vi "RUSHShoot.vi"(1 "In Cluster":T2) -> (0 "Out Cluster":T1)   [LabVIEW 2012]
panel:
  in  "Speed Multiplier":dbl=0.75
  in  "LinReg Adder":dbl=-0.5
  in  "LinReg Multiplier":dbl=0.01
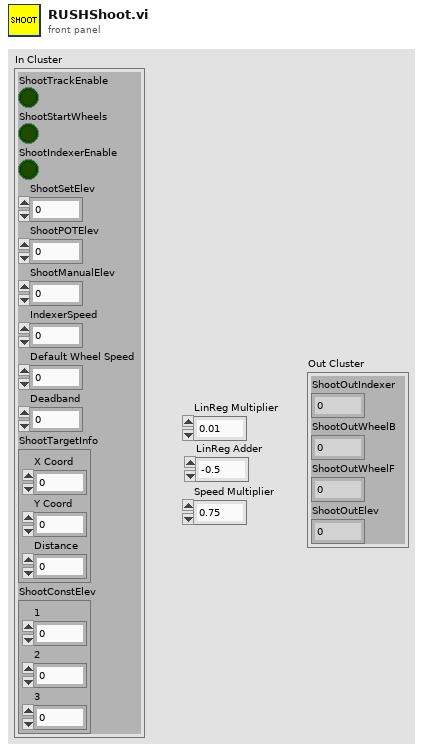
[diagram p1: front panel]
types:
  T1 = cluster{"ShootOutIndexer":dbl, "ShootOutWheelB":dbl, "ShootOutWheelF":dbl, "ShootOutElev":dbl}
  T2 = cluster{"ShootTrackEnable":bool, "ShootStartWheels":bool, "ShootIndexerEnable":bool, "ShootSetElev":dbl, "ShootPOTElev":dbl, "ShootManualElev":dbl, "IndexerSpeed":dbl, "Default Wheel Speed":dbl, "Deadband":dbl, "ShootTargetInfo":cluster{"X Coord":dbl, "Y Coord":dbl, "Distance":dbl}, "ShootConstElev":cluster{"1":dbl, "2":dbl, "3":dbl}}
  T3 = cluster{"X Coord":dbl, "Y Coord":dbl, "Distance":dbl}
  T4 = cluster{"ShootOutIndexer":dbl, "ShootOutWheelB":dbl, "ShootOutWheelF":dbl, "upper limit":dbl}
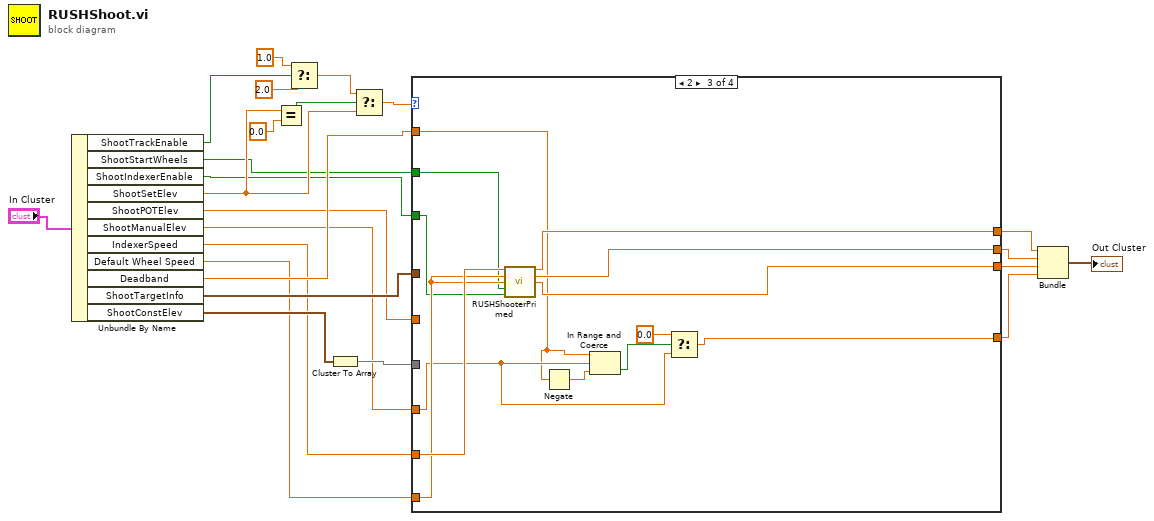
[diagram p0: block diagram]
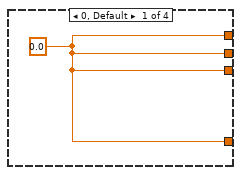
[diagram p2: hidden frame]
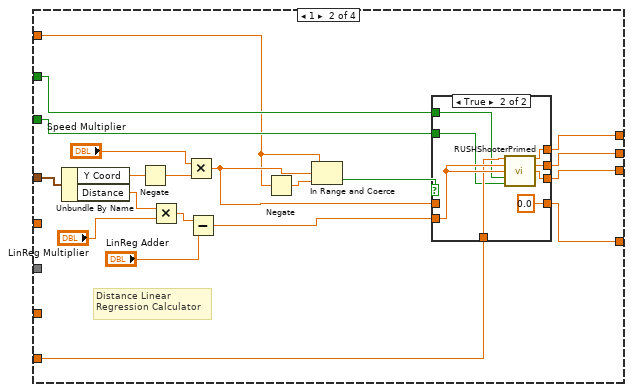
[diagram p3: hidden frame]
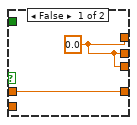
[diagram p4: hidden frame]
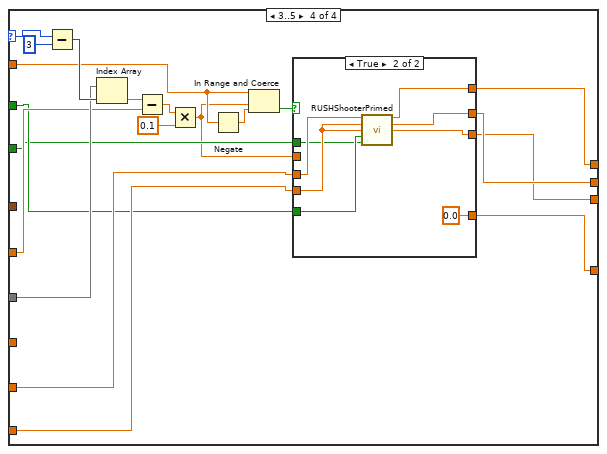
[diagram p5: hidden frame]
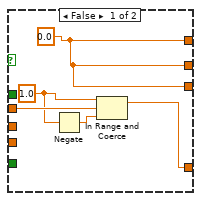
[diagram p6: hidden frame]
diagram:
  n1 = Unbundle By Name("In Cluster") -> ("ShootTrackEnable"=w16:bool, "ShootStartWheels"=w13:bool, "ShootIndexerEnable"=w12:bool, "ShootSetElev"=w15:dbl, "ShootPOTElev"=w10:dbl, "ShootManualElev"=w8:dbl, "IndexerSpeed"=w7:dbl, "Default Wheel Speed"=w6:dbl, "Deadband"=w14:dbl, "ShootTargetInfo"=w11:T3, "ShootConstElev"=w9:cluster{"1":dbl, "2":dbl, "3":dbl})
  n2 = Equal?(x=w15, y=0.0) -> (x = y?=w21:bool)
  n3 = Select(t=1.0, s=w16, f=2.0) -> (s? t:f=w20:dbl)
  n4 = Cluster To Array(cluster=w9) -> (array=w18:dbl[])
  n5 = Select(t=w20, s=w21, f=w15) -> (s? t:f=w19:dbl)
  n6 = case shown="2" w19 {
    selector: w19 -> [_ _ _ w88]
    tunnel: w13 -> [_ w40 w66 w73]
    tunnel: w12 -> [_ w39 w65 w72]
    tunnel: w11 -> [_ w45 _ _]
    tunnel: w10 -> [_ _ _ w83]
    tunnel: w18 -> [_ _ _ w85]
    tunnel: w8 -> [_ _ w58 _]
    tunnel: [w25 w33 w64 w79] -> w5
    tunnel: [w25 w32 w63 w78] -> w4
    tunnel: [w25 w31 w62 w77] -> w3
    tunnel: [w25 w29 w57 w76] -> w2
    tunnel: w7 -> [_ w27 w68 w75]
    tunnel: w6 -> [_ _ w67 w74]
    tunnel: w14 -> [_ w26 w56 w81]
    frame 0, Default {
      w25 = 0.0 ("ShootOutIndexer")
    }
    frame 1 {
      # "Distance Linear\nRegression Calculator"
      n7 = Unbundle By Name(w45) -> ("Y Coord"=w44:dbl, "Distance"=w38:dbl)
      n8 = Negate(x=w44) -> (-x=w43:dbl)
      n9 = Multiply(x=w38, y="LinReg Multiplier") -> (x*y=w36:dbl)
      n10 = Multiply(x="Speed Multiplier", y=w43) -> (x*y=w30:dbl)
      n11 = Subtract(x=w36, y="LinReg Adder") -> (x-y=w34:dbl)
      n12 = Negate(x=w26) -> (-x=w28:dbl)
      n13 = In Range and Coerce(upper limit=w26, x=w30, lower limit=w28) -> (In Range?=w41:bool)  [unwired: 1 out]
      n14 = case shown="True" w41 {
        tunnel: w40 -> [_ w48]
        tunnel: w39 -> [_ w49]
        tunnel: w34 -> [_ w55]
        tunnel: [w47 w54] -> w33
        tunnel: [w47 w53] -> w32
        tunnel: [w47 w52] -> w31
        tunnel: w30 -> [w46 _]
        tunnel: [w46 0.0] -> w29
        tunnel: w27 -> [_ w50]
        frame False {
          w47 = 0.0 ("ShootOutIndexer")
        }
        frame True {
          n15 = call "RUSHShooterPrimed.vi"("IndexerSpeed"=w50, "WheelSpeedF"=w55, "WheelSpeedB"=w55, "ShootStartWheels"=w48, "ShootIndexerEnable"=w49) -> ("ShootOutIndexer"=w54:dbl, "ShootOutWheelB"=w53:dbl, "ShootOutWheelF"=w52:dbl)  [unwired: 8 in]
        }
      }
    }
    frame 2 {
      n16 = call "RUSHShooterPrimed.vi"("IndexerSpeed"=w68, "WheelSpeedF"=w67, "WheelSpeedB"=w67, "ShootStartWheels"=w66, "ShootIndexerEnable"=w65) -> ("ShootOutIndexer"=w64:dbl, "ShootOutWheelB"=w63:dbl, "ShootOutWheelF"=w62:dbl)  [unwired: 8 in]
      n17 = Negate(x=w56) -> (-x=w61:dbl)
      n18 = In Range and Coerce(upper limit=w56, x=w58, lower limit=w61) -> (In Range?=w60:bool)  [unwired: 1 out]
      n19 = Select(t=0.0, s=w60, f=w58) -> (s? t:f=w57:dbl)
    }
    frame 3..5 {
      n20 = Subtract(x=w88, y=3) -> (x-y=w86:i32)
      n21 = Index Array(array=w85, index=w86) -> (element=w84:dbl)
      n22 = Subtract(x=w84, y=w83) -> (x-y=w71:dbl)
      n23 = Multiply(x=w71, y=0.1) -> (x*y=w70:dbl)
      n24 = Negate(x=w81) -> (-x=w82:dbl)
      n25 = In Range and Coerce(upper limit=w81, x=w70, lower limit=w82) -> (In Range?=w80:bool)  [unwired: 1 out]
      n26 = case shown="True" w80 {
        tunnel: [w93 w96] -> w79
        tunnel: [w93 w95] -> w78
        tunnel: [w93 w94] -> w77
        tunnel: w70 -> [w92 _]
        tunnel: [w89 0.0 ("upper limit")] -> w76
        tunnel: w75 -> [_ w100]
        tunnel: w74 -> [_ w99]
        tunnel: w73 -> [_ w98]
        tunnel: w72 -> [_ w97]
        frame False {
          w90 = 1.0 ("upper limit")
          w93 = 0.0
          n27 = Negate(x=w90) -> (-x=w91:dbl)
          n28 = In Range and Coerce(upper limit=w90, x=w92, lower limit=w91) -> (coerced(x)=w89:dbl)  [unwired: 1 out]
        }
        frame True {
          n29 = call "RUSHShooterPrimed.vi"("IndexerSpeed"=w100, "WheelSpeedF"=w99, "WheelSpeedB"=w99, "ShootStartWheels"=w98, "ShootIndexerEnable"=w97) -> ("ShootOutIndexer"=w96:dbl, "ShootOutWheelB"=w95:dbl, "ShootOutWheelF"=w94:dbl)  [unwired: 8 in]
        }
      }
    }
  }
  n30 = Bundle("ShootOutIndexer"=w5, "ShootOutWheelB"=w4, "ShootOutWheelF"=w3, "upper limit"=w2) -> (→"Out Cluster":T4)  [unwired: 1 in]
